vi "New VI Springboard.vi"() -> ()   [LabVIEW 2016]
panel:
  in  "Springboard Name":string
  in  "Cancel":bool
  in  "OK":bool caption="OK2"
  # "Choose the Name for Your New Springboard"
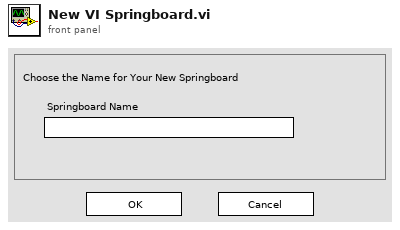
[diagram p1: front panel]
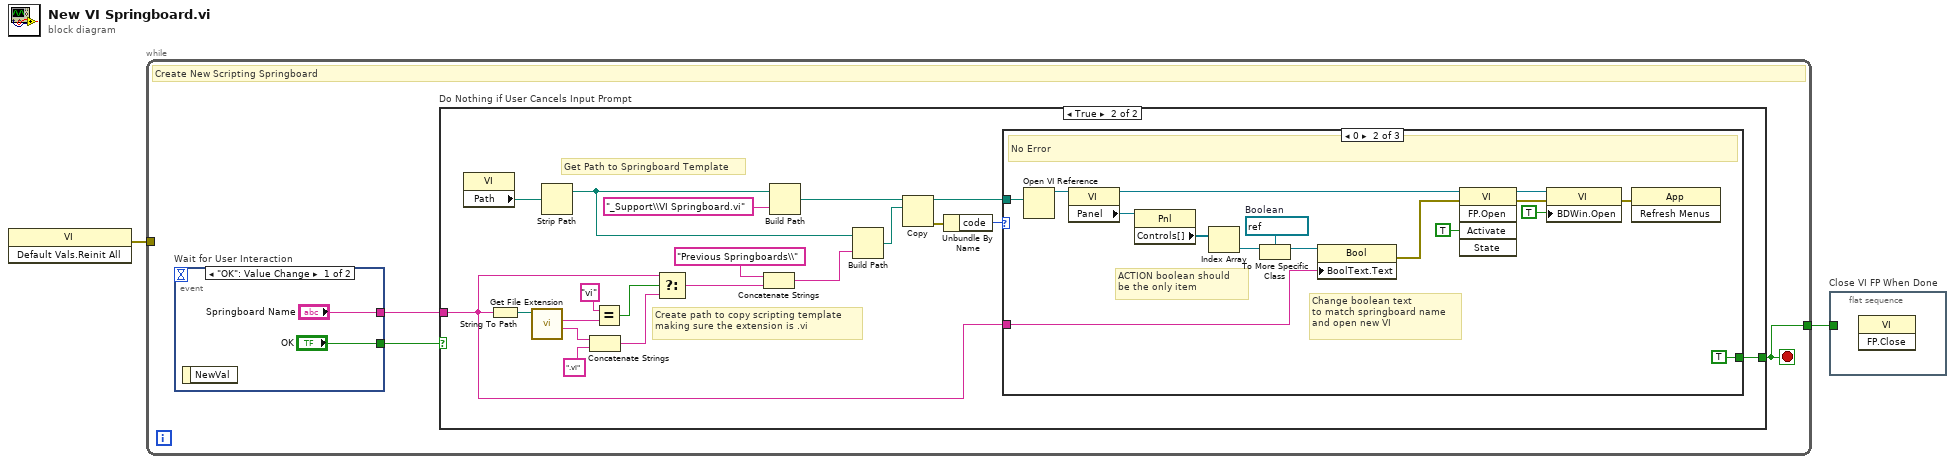
[diagram p0: block diagram]
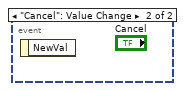
[diagram p2: hidden frame]
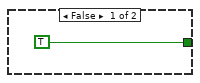
[diagram p3: hidden frame]
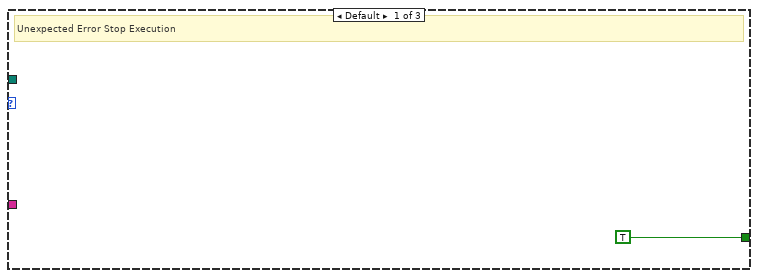
[diagram p4: hidden frame]
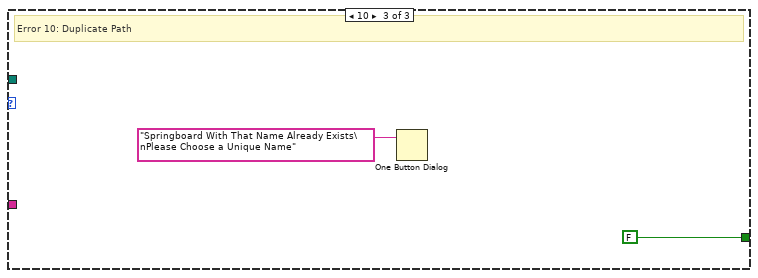
[diagram p5: hidden frame]
diagram:
  n1 = invoke class="VI" method="Default Vals.Reinit All"() -> (error out=w2:errorcluster)  [unwired: 3 in, 2 out]
  n2 = while {
    tunnel: w2 -> [_]
    tunnel: [w3] -> w1
    stop <- w3 stop-if-true
    # "Create New Scripting Springboard"
    n3 = event "Wait for User Interaction" shown="[0] \"OK\": Value Change" {
      selector: _ -> [_ _]
      dyn-events: _ -> [_ _]
      timeout: _ -> [_ _]
      tunnel: ["OK" _] -> w5
      tunnel: ["Springboard Name" _] -> w4
      event "OK": Value Change {
        n4 = event-data() -> ()  [unwired: 1 in, 1 out]
      }
      event "Cancel": Value Change {
        n5 = event-data() -> ()  [unwired: 1 in, 1 out]
      }
    }
    n6 = case "Do Nothing if User Cancels Input Prompt" shown="True" w5 {
      tunnel: w4 -> [_ w9]
      tunnel: [TRUE w10] -> w3
      frame False {
      }
      frame True {
        # "Create path to copy scripting template making sure the extension is .vi"
        # "Get Path to Springboard Template"
        n7 = property class="VI"() -> ("Path"=w28:path)  [unwired: 2 in, 2 out]
        n8 = String To Path(string=w9) -> (path=w22:path)
        n9 = call <vilib>:"Get File Extension.vi"("file"=w22) -> ("filename without extension"=w18:string, "lowercase file extension"=w21:string)  [unwired: 6 in, 3 out]
        n10 = Strip Path(path=w28) -> (stripped path=w25:path)  [unwired: 1 out]
        n11 = Concatenate Strings(w18, ".vi" ("string")) -> (w16:string)
        n12 = Equal?(x="vi" ("y"), y=w21) -> (x = y?=w19:bool)
        n13 = Select(t=w9, s=w19, f=w16) -> (s? t:f=w15:string)
        n14 = Concatenate Strings("Previous Springboards\\" ("name or relative path"), w15) -> (w14:string)
        n15 = Build Path(base path=w25, name or relative path="_Support\\VI Springboard.vi") -> (appended path=w26:path)
        n16 = Build Path(base path=w25, name or relative path=w14) -> (appended path=w23:path)
        n17 = Copy(10:w23, 11:w26) -> (0:w13:errorcluster, 3:w11:path)  [unwired: 3 in, 1 out]
        n18 = Unbundle By Name(w13) -> ("code"=w12:i32)
        n19 = case shown="0" w12 {
          tunnel: w11 -> [_ w45 _]
          tunnel: [TRUE TRUE FALSE] -> w10
          tunnel: w9 -> [_ w37 _]
          frame Default {
            # "Unexpected Error Stop Execution"
          }
          frame 0 {
            w39 = refnum<vi> refnum  # Boolean
            # "Change boolean text\nto match springboard name\nand open new VI"
            # "ACTION boolean should\nbe the only item"
            # "No Error"
            n20 = Open VI Reference(vi path=w45) -> (vi reference=w43:refnum<vi>)  [unwired: 5 in, 1 out]
            n21 = property class="VI"(reference=w43) -> (reference out=w36:refnum<vi>, "Panel"=w42:refnum<vi>)  [unwired: 1 in, 1 out]
            n22 = property class="Pnl"(reference=w42) -> ("Controls[]"=w41:refnum<vi>[])  [unwired: 1 in, 2 out]
            n23 = Index Array(array=w41) -> (element=w40:refnum<vi>)  [unwired: 1 in]
            n24 = To More Specific Class(target class=w39, reference=w40) -> (specific class reference=w38:refnum<vi>)  [unwired: 1 in, 1 out]
            n25 = property class="Bool"(reference=w38, "BoolText.Text"=w37) -> (error out=w35:errorcluster)  [unwired: 1 in, 1 out]
            n26 = invoke class="VI" method="FP.Open"(reference=w36, error in=w35, "Activate"=TRUE ("Activate?")) -> (reference out=w31:refnum<vi>, error out=w33:errorcluster)  [unwired: 2 in, 3 out]
            n27 = property class="VI"(reference=w31, error in=w33, "BDWin.Open"=TRUE ("Activate?")) -> (error out=w32:errorcluster)  [unwired: 1 out]
            n28 = invoke class="App" method="Refresh Menus"(error in=w32) -> ()  [unwired: 2 in, 3 out]
          }
          frame 10 {
            # "Error 10: Duplicate Path"
            n29 = One Button Dialog(message="Springboard With That Name Already Exists\nPlease Choose a Unique Name") -> ()  [unwired: 1 in, 1 out]
          }
        }
      }
    }
  }
  n30 = flat-sequence "Close VI FP When Done" {
    tunnel: w1 -> [_]
    frame #0 {
      n31 = invoke class="VI" method="FP.Close"() -> ()  [unwired: 3 in, 3 out]
    }
  }
